vi "tool_Unicode_Convert ASCII to Unicode (1D).vi"(4 "ASCII":string[](array[string])) -> (1 "Unicode":string[](array[string]))   [LabVIEW 2020]
uses:
  kernel32.dll
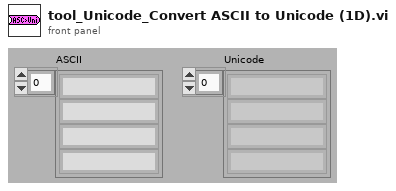
[diagram p1: front panel]
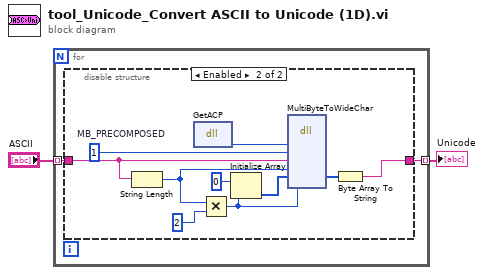
[diagram p0: block diagram]
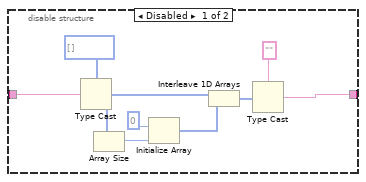
[diagram p2: hidden frame]
diagram:
  n1 = for {
    tunnel: "ASCII" -> [w4] mode=indexing
    tunnel: [w3] -> w1 mode=indexing
    n2 = disable-structure shown="Enabled" {
      disable-tunnel: w4 -> [w13 w16]
      disable-tunnel: [w5 w15] -> w3
      frame Disabled {
        n3 = Type Cast(type=u8[] [], x=w13) -> (*(type *) &x=w9:u8[])
        n4 = Array Size(array=w9) -> (size(s)=w11:i32)
        n5 = Initialize Array(u8 0, w11) -> (w8:u8[])
        n6 = Interleave 1D Arrays(w9, w8) -> (w7:u8[])
        n7 = Type Cast(type="", x=w7) -> (*(type *) &x=w5:string)
      }
      frame Enabled {
        w22 = u32 1  # MB_PRECOMPOSED
        n8 = String Length(string=w16) -> (length=w14:i32)
        n9 = dll-call lib="kernel32.dll" fn="GetACP" label="GetACP()"() -> (w17:u32)  [unwired: 3 in, 2 out]
        n10 = Multiply(x=w14, y=2) -> (x*y=w18:i32)
        n11 = Initialize Array(u8 0, w18) -> (w20:u8[])
        n12 = dll-call lib="kernel32.dll" fn="MultiByteToWideChar"("codePage"=w17, "dwFlags"=w22, "pMultiByteStr"=w16, "cbMultiByte"=w14, "lpWideCharStr"=w20, "cchWideChar"=w18) -> ("lpWideCharStr"=w19:u8[])  [unwired: 8 in, 3 out]
        n13 = Byte Array To String(unsigned byte array=w19) -> (string=w15:string)
      }
    }
  }
  "Unicode" <- w1
